vi "AB Status 2 AB Display Status.vi"(10 "Autobalance Status In":T1[](array[typedef])) -> (2 "Autobalance Statuses Out":T5[](array[typedef]))   [LabVIEW 2013]
uses:
  Autobalance Display Data Point.ctl
  Autobalance Stage.ctl
  Apps/Yes No Button.ctl
  Autobalance Status Data.ctl
  Autobalance Data Point.ctl
panel:
  # "Cmd"
  # "Servo"
  # "Cmd"
  # "Servo"
  # "Cmd"
  # "Servo Error"
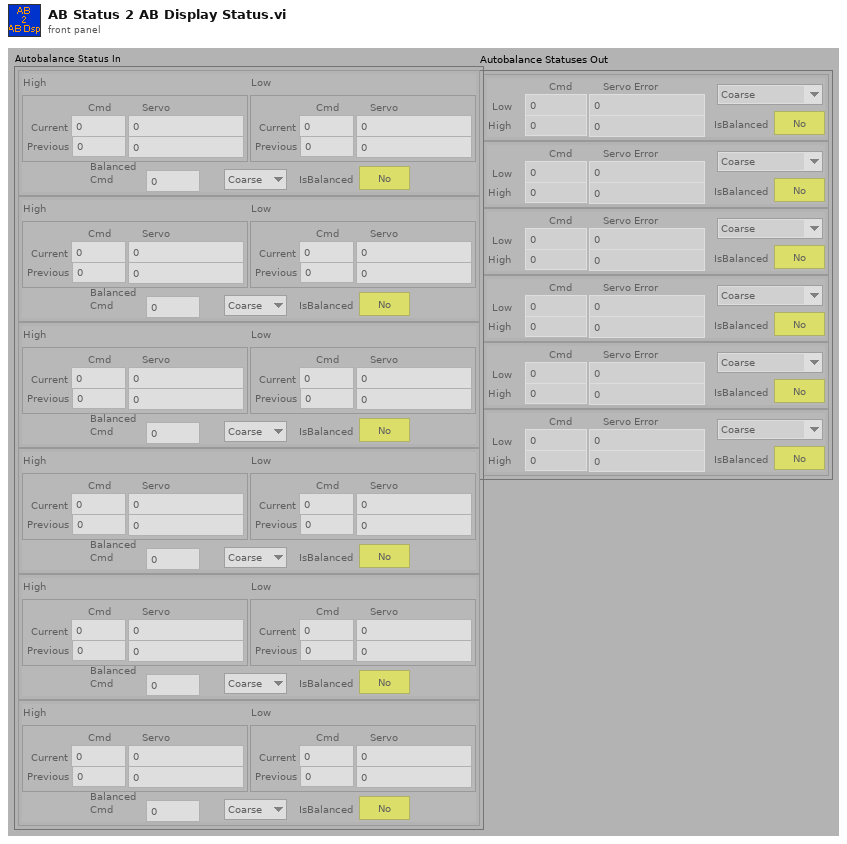
[diagram p1: front panel]
types:
  T1 = typedef "Autobalance Status Data.ctl" = cluster{"IsBalanced":T2, "Autobalance Stage":T3, "High":T4, "Low":T4, "Balanced \nCmd":dbl}
  T2 = typedef "Yes No Button.ctl" = bool
  T3 = typedef "Autobalance Stage.ctl" = enum16{"Coarse", "Fine", "Backing Up", "Done"}
  T4 = typedef "Autobalance Data Point.ctl" = cluster{"cCmd":dbl, "cServo":dbl, "pCmd":dbl, "pServo":dbl}
  T5 = typedef "Autobalance Display Data Point.ctl" = cluster{"LoCmd":dbl, "LoServo":dbl, "HiCmd":dbl, "HiServo":dbl, "Autobalance Stage":T3, "IsBalanced":T2}
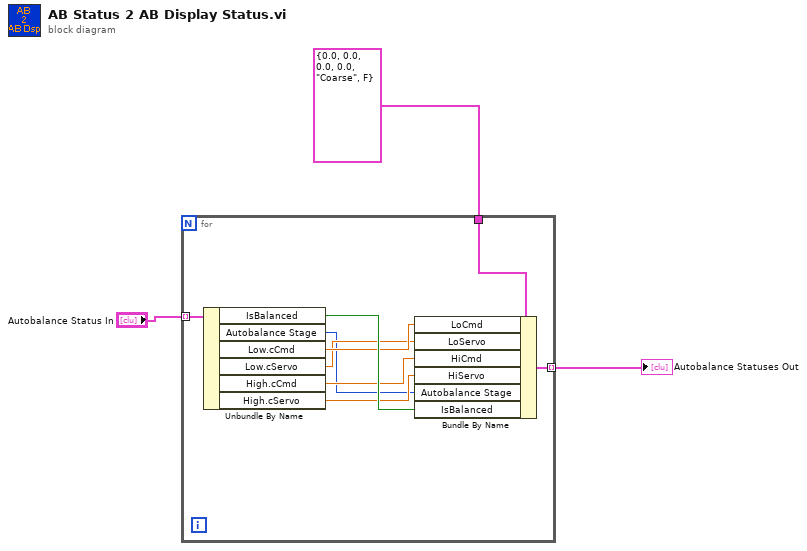
[diagram p0: block diagram]
diagram:
  n1 = for {
    tunnel: "Autobalance Status In" -> [w12] mode=indexing
    tunnel: T5 {"LoCmd"=0.0, "LoServo"=0.0, "HiCmd"=0.0, "HiServo"=0.0, "Autobalance Stage"=enum."Coarse", "IsBalanced"=FALSE} ("Autobalance Diplsay Data Point") -> [w11]
    tunnel: [w4] -> w1 mode=indexing
    n2 = Unbundle By Name(w12) -> ("IsBalanced"=w10:T2, "Autobalance Stage"=w5:T3, "Low.cCmd"=w9:dbl, "Low.cServo"=w8:dbl, "High.cCmd"=w7:dbl, "High.cServo"=w6:dbl)
    n3 = Bundle By Name(cluster=w11, "LoCmd"=w9, "LoServo"=w8, "HiCmd"=w7, "HiServo"=w6, "Autobalance Stage"=w5, "IsBalanced"=w10) -> (w4:T5)
  }
  "Autobalance Statuses Out" <- w1
